vi "Get Marker Polarity.vi"(8 "error in (no error)":errorcluster {"code" format="%.0x"}, 9 "MarkerIndex (Ss Digital Modulation Arb Marker Index One)":i32(ring) items=["Ss Digital Modulation Arb Marker Index One", "Ss Digital Modulation Arb Marker Index Two", "Ss Digital Modulation Arb Marker Index Three", "Ss Digital Modulation Arb Marker Index Four", "Ss Digital Modulation Arb Marker Index All", "Ss Digital Modulation Arb Marker Index None"], 11 "instrument handle":refnum<k15>) -> (0 "error out":errorcluster {"code" format="%.0x"}, 2 "Val":i32, 3 "instrument handle out":refnum<k15>)   [LabVIEW 2009, in "Keysight XSAn.lvlib"]
doc: "Get the polarity of marker.\n\nSupported Models: M8920A, M9420A, M9421A."
uses:
  <instrlib>/Keysight XSAn/Keysight XSAn.lvlib
  AgXSAn.dll
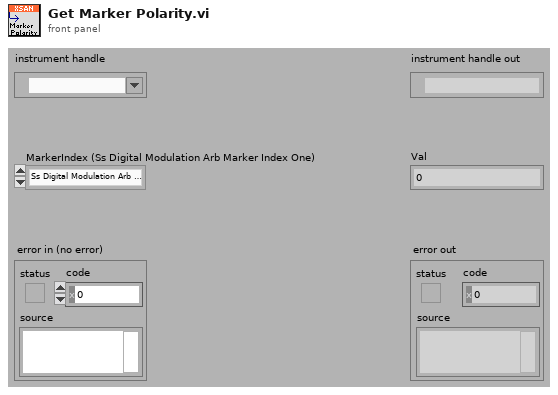
[diagram p1: front panel]
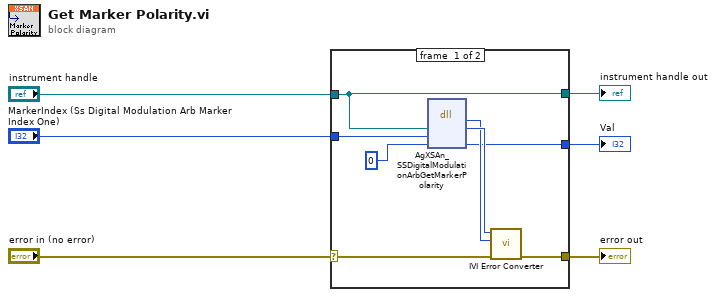
[diagram p0: block diagram]
diagram:
  n1 = case shown="No Error" "error in (no error)" {
    selector: "error in (no error)" -> [w12 w16]
    tunnel: [w11 w16] -> w6
    tunnel: "instrument handle" -> [w7 w15]
    tunnel: "MarkerIndex (Ss Digital Modulation Arb Marker Index One)" -> [w10 _]
    tunnel: [w8 _] -> w2
    tunnel: [w7 w15] -> w1
    frame #0 {
      n2 = dll-call lib="AgXSAn**.dll" fn="AgXSAn_SSDigitalModulationArbGetMarkerPolarity"("Vi"=w7, "MarkerIndex"=w10, "Val"=0) -> ("return type"=w13:i32, "Vi"=w14:u32, "Val"=w8:i32)  [unwired: 4 in, 2 out]
      n3 = call <instrlib>:"IVI Error Converter.vi"("error in (no error)"=w12, "IVI error code (0)"=w13, "instrument handle"=w14) -> ("error out"=w11:errorcluster)  [unwired: 7 in, 1 out]
    }
    frame #1 {
    }
  }
  "error out" <- w6
  "instrument handle out" <- w1
  "Val" <- w2
